vi "RichToFlatnidaqmx_grpc_StopTaskRequest.vi"(5 "OutputClusterType":T1, 11 "InputCluster":T3) -> (3 "OutputCluster":T1)   [LabVIEW 2021, in "NI_DAQmx_client.lvlib"]
uses:
  NI_DAQmx_client.lvlib
  nidaqmx_grpc_StopTaskRequest.ctl
  nidevice_grpc_Session_session/nidevice_grpc_Session_session.lvclass
  nidevice_grpc_Session.ctl
  nidaqmx_grpc_StopTaskRequest_Flat.ctl
  nidevice_grpc_Session_Flat.ctl
  nidevice_grpc_Session_session/nidevice_grpc_Session_session.lvclass/nidevice_grpc_Session_session.ctl
  nidevice_grpc_Session_session/GetActiveFieldIndex.vi
  nidevice_grpc_Session_session/Getname.vi
  nidevice_grpc_Session_session/Getid.vi
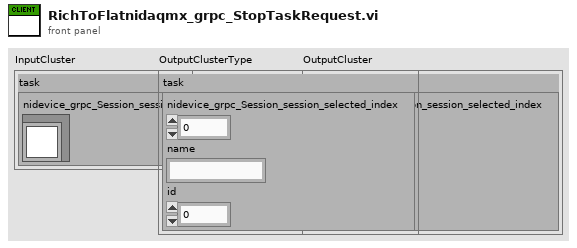
[diagram p1: front panel]
types:
  T1 = typedef "NI_DAQmx_client.lvlib/nidaqmx_grpc_StopTaskRequest_Flat.ctl" = cluster{"task":T2}
  T2 = typedef "NI_DAQmx_client.lvlib/nidevice_grpc_Session_Flat.ctl" = cluster{"nidevice_grpc_Session_session_selected_index":i32, "name":string, "id":u32}
  T3 = typedef "NI_DAQmx_client.lvlib/nidaqmx_grpc_StopTaskRequest.ctl" = cluster{"task":T4}
  T4 = typedef "NI_DAQmx_client.lvlib/nidevice_grpc_Session.ctl" = cluster{"nidevice_grpc_Session_session":refnum<class "nidevice_grpc_Session_session.lvclass">}
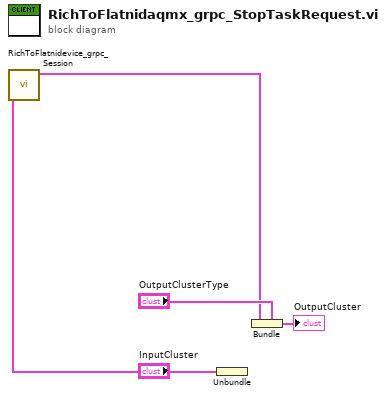
[diagram p0: block diagram]
diagram:
  n1 = Unbundle "Unbundle"("InputCluster") -> ("task"=w2:T4)
  n2 = call "RichToFlatnidevice_grpc_Session.vi"("InputCluster"=w2) -> ("OutputCluster"=w1:T2)  [unwired: 10 in]
  n3 = Bundle "Bundle"(cluster="OutputClusterType", "task"=w1) -> (→"OutputCluster":T1)
